vi "Clear Error For Attach and Close.vi"(8 "error in":errorcluster, 11 "instrument initialize and close session behavior":T1) -> (0 "error out":errorcluster)   [LabVIEW 2020, in "MeasurementLink Session Management V1.lvlib" / "Session Reservation.lvclass"]
uses:
  Session Reservation.lvclass
  MeasurementLink Instrument/ISession Factory/Initialize and Close Session Behavior.ctl
  Session Reservation.lvclass/Session Reservation.ctl
  MeasurementLink Instrument/ISession Factory/ISession Factory.lvclass
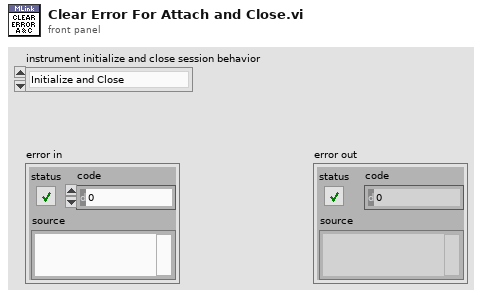
[diagram p1: front panel]
types:
  T1 = typedef "MeasurementLink Instrument.lvlib/ISession Factory.lvclass/Initialize and Close Session Behavior.ctl" = enum16{"Initialize and Close", "Attach and Detach", "Initialize and Detach", "Attach and Close"}
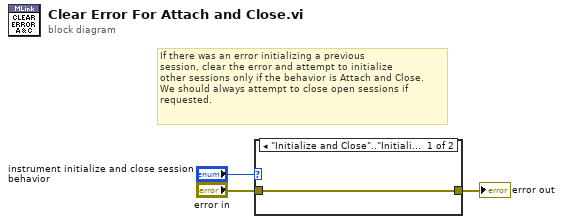
[diagram p0: block diagram]
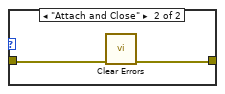
[diagram p2: hidden frame]
diagram:
  # "If there was an error initializing a previous\nsession, clear the error and attempt to initialize\nother sessions only if the behavior is Attach and Close.\nWe should always attempt to close open sessions if \nrequested."
  n1 = case shown="\"Initialize and Close\"..\"Initialize and Detach\"" "instrument initialize and close session behavior" {
    tunnel: "error in" -> [w4 w6]
    tunnel: [w4 w5] -> w1
    frame "Initialize and Close".."Initialize and Detach" {
    }
    frame "Attach and Close" {
      n2 = call <vilib>:"Clear Errors.vi"("error in (no error)"=w6) -> ("error out"=w5:errorcluster)  [unwired: 5 in, 1 out]
    }
  }
  "error out" <- w1
